vi "Advance past Line Ending.vi"(9 "Offset":i32, 11 "JSON":u8[](array[numeric]) format="%.0x") -> (1 "Offset after Line Ending":i32)   [LabVIEW 2019, in "JSONtext.lvlib"]
uses:
  JSONtext.lvlib
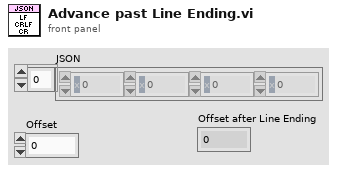
[diagram p1: front panel]
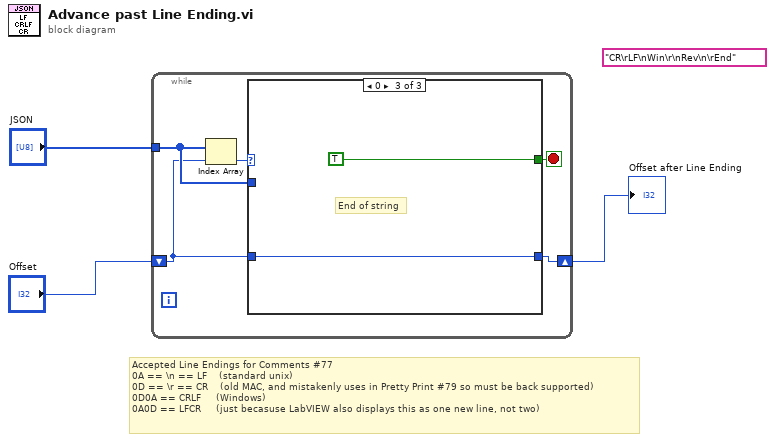
[diagram p0: block diagram]
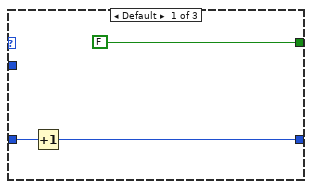
[diagram p2: hidden frame]
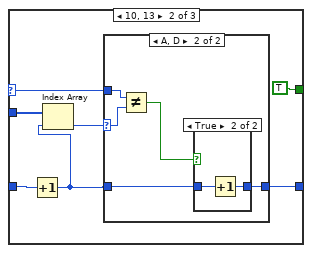
[diagram p3: hidden frame]
diagram:
  (unwired) "CR\rLF\nWin\r\nRev\n\rEnd"
  # "Accepted Line Endings for Comments #77\n0A == \\n == LF    (standard unix)\n0D == \\r == CR    (old MAC, and mistakenly uses in Pretty Print #79 so must be back supported)\n0D0A == CRLF     (Windows)\n0A0D == LFCR     (just becasuse LabVIEW also displays this as one new line, not two)"
  n1 = while {
    tunnel: "JSON" -> [w5]
    shift-right: [w6] -> w2
    shift-left: "Offset" -> [w4]
    stop <- w7 stop-if-true
    n2 = Index Array(array=w5, index=w4) -> (element=w8:u8)
    n3 = case shown="0" w8 {
      selector: w8 -> [_ w14 _]
      tunnel: w4 -> [w10 w13 w29]
      tunnel: [FALSE TRUE TRUE] -> w7
      tunnel: [w9 w16 w29] -> w6
      tunnel: w5 -> [_ w17 _]
      frame Default {
        n4 = Increment(x=w10) -> (x+1=w9:i32)
      }
      frame 10, 13 {
        n5 = Increment(x=w13) -> (x+1=w12:i32)
        n6 = Index Array(array=w17, index=w12) -> (element=w15:u8)
        n7 = case shown="A, D" w15 {
          selector: w15 -> [_ w21]
          tunnel: w12 -> [w19 w24]
          tunnel: [w19 w23] -> w16
          tunnel: w14 -> [_ w20]
          frame 0, Default {
          }
          frame 10, 13 {
            n8 = Not Equal?(x=w20, y=w21) -> (x != y?=w22:bool)
            n9 = case shown="True" w22 {
              tunnel: w24 -> [w25 w27]
              tunnel: [w25 w26] -> w23
              frame False {
              }
              frame True {
                n10 = Increment(x=w27) -> (x+1=w26:i32)
              }
            }
          }
        }
      }
      frame 0 {
        # "End of string"
      }
    }
  }
  "Offset after Line Ending" <- w2
